vi "ShiftRegister-Simple.vi"() -> ()   [LabVIEW 2020]
doc: "Use this template to create an application that executes repeatedly until you click the Stop button. This template polls the state of the Stop button and does not use events. Use the Top-Level Application template (not available in the Base package) to create a single-loop application with event handling."
panel:
  in  "Write Data":dbl
  out "Data Read":dbl
  in  "Operate":enum16{"Read", "Write"}(ring)
  out "error out":errorcluster
  in  "error in":errorcluster
  in  "stop":bool
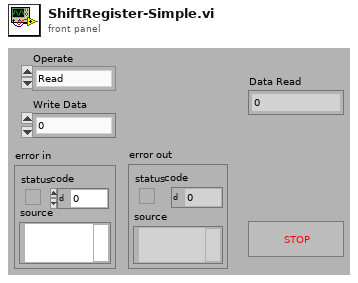
[diagram p1: front panel]
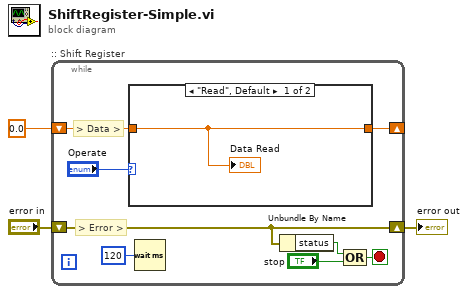
[diagram p0: block diagram]
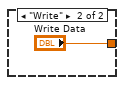
[diagram p2: hidden frame]
diagram:
  n1 = while ":: Shift Register" {
    shift-right: [w8] -> _
    shift-left: 0.0 ("Write Data") -> [w9]
    shift-right: [w11] -> w2
    shift-left: "error in" -> [w11]
    stop <- w5 stop-if-true
    # "> Data >"
    # "> Error >"
    n2 = case shown="\"Read\", Default" "Operate" {
      tunnel: w9 -> [w12 _]
      tunnel: [w12 "Write Data"] -> w8
      frame "Read", Default {
        "Data Read" <- w12
      }
      frame "Write" {
      }
    }
    n3 = Wait (ms)(milliseconds to wait=u32 120) -> ()  [unwired: 1 out]
    n4 = Unbundle By Name(w11) -> ("status"=w7:bool)
    n5 = Compound Arithmetic op=OR(w7, "stop") -> (w5:bool)
  }
  "error out" <- w2
